vi "LMS_EnableChannel.vi"(0 "device_In":i64, 5 "dir_tx":u8, 7 "chan":u64, 11 "error in (no error)":errorcluster, 12 "enabled":i8) -> (4 "device_Out":i64, 15 "error out":errorcluster)   [LabVIEW 2013, in "LMS_LV_Drv.lvlib"]
uses:
  LMS_LV_Drv.lvlib
  LimeSuite.dll
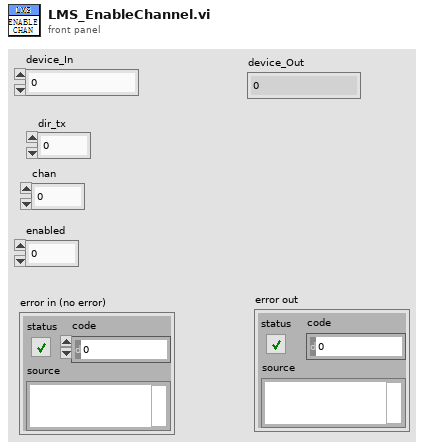
[diagram p1: front panel]
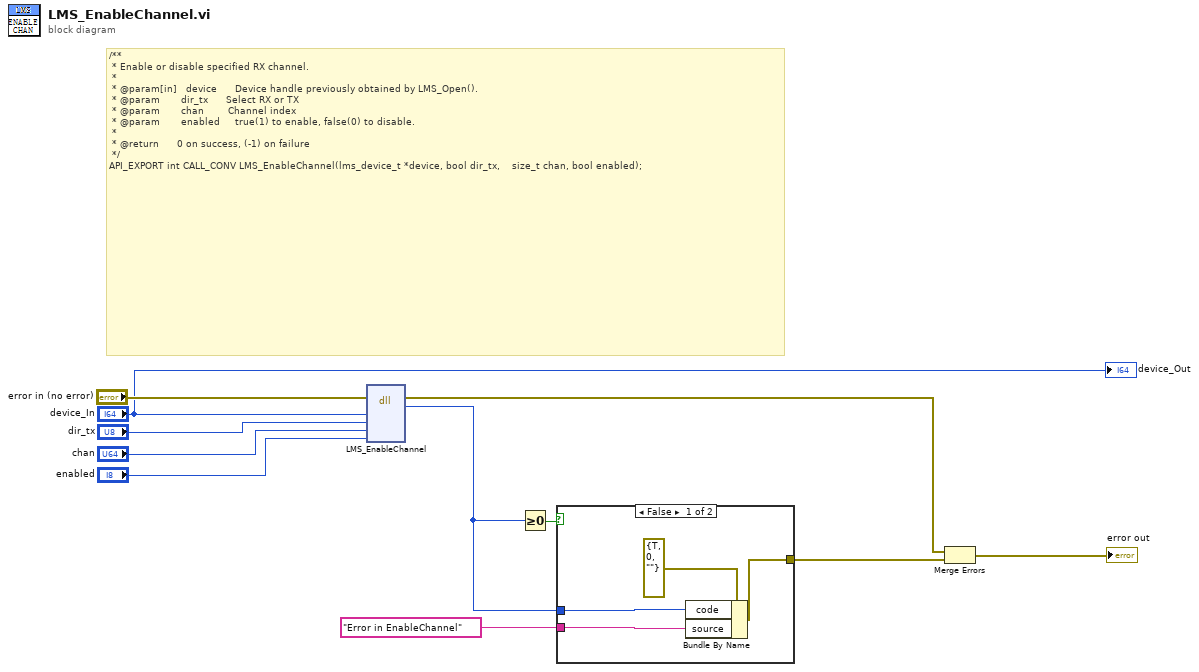
[diagram p0: block diagram]
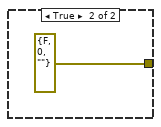
[diagram p2: hidden frame]
diagram:
  # "/**\n * Enable or disable specified RX channel.\n *\n * @param[in]   device      Device handle previously obtained by LMS_Open().\n * @param       dir_tx      Select RX or TX\n * @param       chan        Channel index\n * @param       enabled     true(1) to enable, false(0) to disable.\n *\n * @return      0 on success, (-1) on failure\n */\nAPI_EXPORT int CALL_CONV LMS_EnableChannel(lms_device_t *device, bool dir_tx,    size_t chan, bool enabled);"
  n1 = dll-call lib="PTH1mabs CUsersOTADesktop书籍出版程序8.第八章LimeSDR_LabVIEW_Driver-master\nLimeSuite.dll" fn="LMS_EnableChannel"(error in="error in (no error)", "device"="device_In", "dir_tx"="dir_tx", "chan"="chan", "enabled"="enabled") -> (error out=w3:errorcluster, "return type"=w1:i32)  [unwired: 6 in, 1 out]
  n2 = Greater Or Equal To 0?(x=w1) -> (x >= 0?=w6:bool)
  n3 = case shown="False" w6 {
    tunnel: [w14 errorcluster {"status"=FALSE, "code"=0, "source"=""} ("error in")] -> w4
    tunnel: w1 -> [w13 _]
    tunnel: "Error in EnableChannel" ("source") -> [w12 _]
    frame False {
      n4 = Bundle By Name(cluster=errorcluster {"status"=TRUE, "code"=0, "source"=""} ("error in"), "code"=w13, "source"=w12) -> (w14:errorcluster)
    }
    frame True {
    }
  }
  n5 = Merge Errors(w3, w4) -> (→"error out":errorcluster)
  "device_Out" <- "device_In"
